vi "Update.vi"(6 "Engine in":refnum<class "Engine.lvclass">, 7 "CursorIn":refnum<class "RT_Sprite.lvclass">, 8 "error in (no error)":errorcluster, 10 "Game(readonly)":refnum<class "Game.lvclass">, 11 "GameMenu in":refnum<class "GameMenu.lvclass">) -> (0 "error out":errorcluster, 1 "State":T1, 3 "GameMenu out":refnum<class "GameMenu.lvclass">, 4 "Engine out":refnum<class "Engine.lvclass">, 5 "CursorOut":refnum<class "RT_Sprite.lvclass">)   [LabVIEW 2019, in "RT_Game.lvlib" / "GameMenu.lvclass"]
uses:
  GameMenu.lvclass
  Menu/States.ctl
  RT_Sprite/RT_Sprite.lvclass
  C:/Users/FreshBob/Dropbox/VIs/myRIO_GameConsole/RT/RT_Game/GameObject/GameObject.lvclass
  Game/Game.lvclass
  Engine/Engine.lvclass
  GameMenu.lvclass/GameMenu.ctl
  Game/Game.lvclass/Game.ctl
  Engine/Coordinate.ctl
  Engine/Engine.lvclass/Engine.ctl
  Game/Read State.vi
  Engine/Read Controls.vi
  Game/Read Singleplayer.vi
  GameObject/GameObject.lvclass
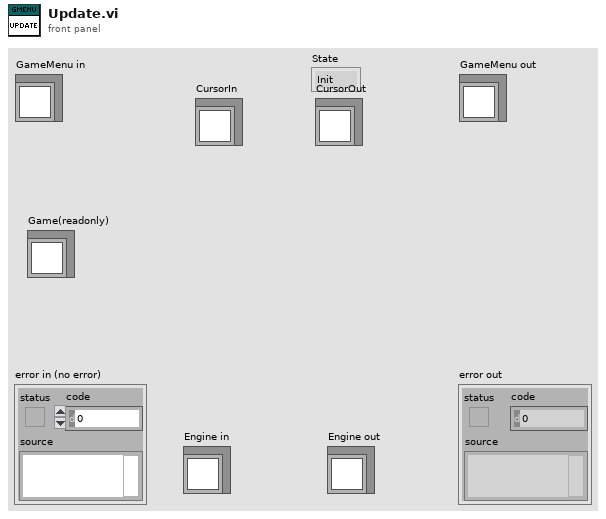
[diagram p1: front panel]
types:
  T1 = typedef "RT_Game.lvlib/Game.lvclass/States.ctl" = enum16{"Init", "Restart", "Menu", "Game", "Resume", "ToggleSingleplayer", "LoadNextGame", "ExitToMenu", "NewHighscore", "GameOver", "SlideOut", "FadeToMenu", "StartFadeToMenu"}
  T2 = typedef "RT_Game.lvlib/Engine.lvclass/Coordinate.ctl" = cluster{"x":dbl, "y":dbl}
  T3 = typedef "RT_Game.lvlib/Game.lvclass/Controls.ctl" = cluster{"Controls_1":T4, "Controls_2":cluster{"DirectionX":i8, "DirectionY":i8, "Button1":bool, "Button2":bool}, "SystemButton":bool}
  T4 = typedef "RT_Game.lvlib/Game.lvclass/ControlPlayer.ctl" = cluster{"DirectionX":i8, "DirectionY":i8, "Button1":bool, "Button2":bool}
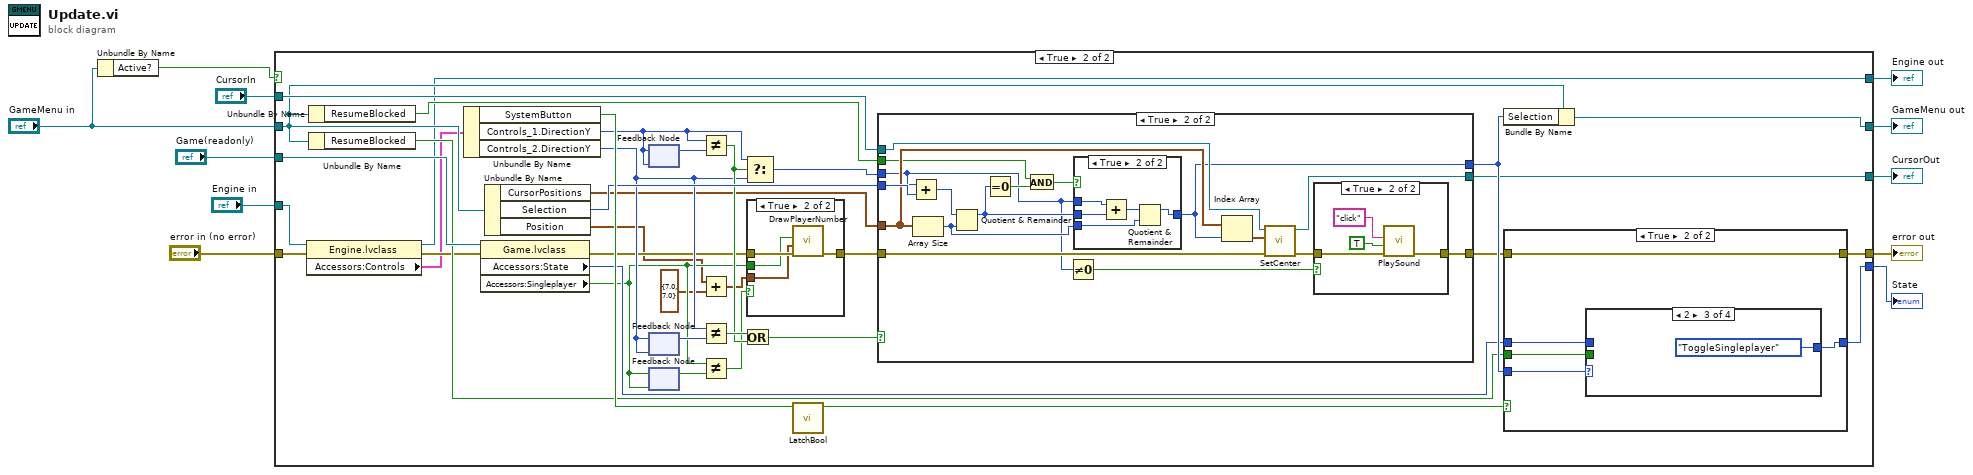
[diagram p0: block diagram]
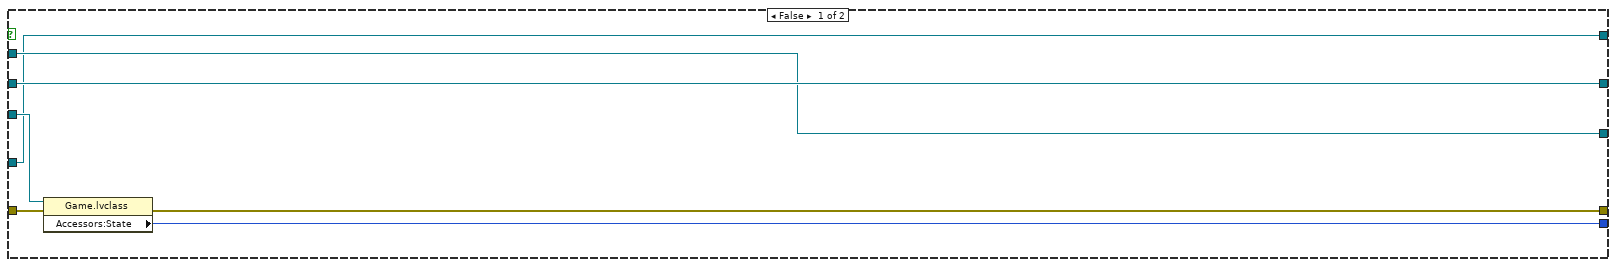
[diagram p2: hidden frame]
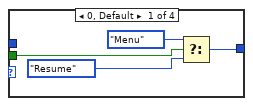
[diagram p8: hidden frame]
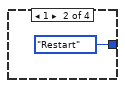
[diagram p9: hidden frame]
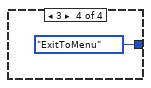
[diagram p10: hidden frame]
diagram:
  n1 = Unbundle By Name("GameMenu in") -> ("Active?"=w8:bool)
  n2 = case shown="True" w8 {
    tunnel: [w16 w54] -> w11
    tunnel: "error in (no error)" -> [w15 w40]
    tunnel: [w13 w52] -> w9
    tunnel: "GameMenu in" -> [w18 w24]
    tunnel: [w18 w36] -> w6
    tunnel: "CursorIn" -> [w17 w41]
    tunnel: [w17 w39] -> w4
    tunnel: "Game(readonly)" -> [w14 w34]
    tunnel: "Engine in" -> [w12 w21]
    tunnel: [w12 w19] -> w1
    frame False {
      n3 = property class="Game.lvclass"(reference=w14, error in=w15) -> (error out=w16:errorcluster, "Accessors:State"=w13:T1)  [unwired: 1 out]
    }
    frame True {
      n4 = property class="Engine.lvclass"(reference=w21, error in=w40) -> (reference out=w19:refnum<class "Engine.lvclass">, error out=w22:errorcluster, "Accessors:Controls"=w20:T3)
      n5 = Unbundle By Name(w24) -> ("ResumeBlocked"=w25:bool)
      n6 = Unbundle By Name(w24) -> ("ResumeBlocked"=w23:bool)
      n7 = Unbundle By Name(w20) -> ("SystemButton"=w55:bool, "Controls_1.DirectionY"=w44:i8, "Controls_2.DirectionY"=w43:i8)
      n8 = property class="Game.lvclass"(reference=w34, error in=w22) -> (error out=w35:errorcluster, "Accessors:State"=w33:T1, "Accessors:Singleplayer"=w29:bool)  [unwired: 1 out]
      n9 = Unbundle By Name(w24) -> ("CursorPositions"=w37:T2[], "Selection"=w50:i16, "Position"=w28:T2)
      n10 = feedback-in #1(w44) -> ()
      n11 = feedback #1(w44) -> (w51:i8)
      n12 = feedback #2(w43) -> (w49:i8)
      n13 = feedback-in #2(w43) -> ()
      n14 = feedback-in #3(w29) -> ()
      n15 = feedback #3(w29) -> (w32:bool)
      n16 = Not Equal?(x=w44, y=w51) -> (x != y?=w45:bool)
      n17 = Add(x=w28, y=T2 {"x"=7.0, "y"=7.0}) -> (x+y=w26:T2)
      n18 = Not Equal?(x=w43, y=w49) -> (x != y?=w47:bool)
      n19 = Not Equal?(x=w29, y=w32) -> (x != y?=w30:bool)
      n20 = Or(x=w47, y=w45) -> (x .or. y?=w48:bool)
      n21 = Select(t=w44, s=w45, f=w43) -> (s? t:f=w46:i8)
      n22 = case shown="True" w30 {
        tunnel: w35 -> [w56 w60]
        tunnel: [w56 w59] -> w31
        tunnel: w29 -> [_ w58]
        tunnel: w26 -> [_ w57]
        frame False {
        }
        frame True {
          n23 = call "DrawPlayerNumber.vi"("error in (no error)"=w60, "Position"=w57, "Accessors:Singleplayer"=w58) -> ("error out"=w59:errorcluster)  [unwired: 8 in]
        }
      }
      n24 = call "LatchBool.vi"("Boolean"=w55) -> ("Latched Boolean"=w53:bool)  [unwired: 10 in]
      n25 = case shown="True" w48 {
        tunnel: w50 -> [w63 w80]
        tunnel: [w63 w71] -> w42
        tunnel: w46 -> [_ w65]
        tunnel: w41 -> [w61 w76]
        tunnel: w31 -> [w62 w79]
        tunnel: [w61 w75] -> w39
        tunnel: [w62 w66] -> w38
        tunnel: w37 -> [_ w78]
        tunnel: w25 -> [_ w67]
        frame False {
        }
        frame True {
          n26 = Add(x=w65, y=w80) -> (x+y=w73:i16)
          n27 = Array Size(array=w78) -> (size(s)=w72:i32)
          n28 = Quotient & Remainder(x=w73, y=w72) -> (x-y*floor(x/y)=w70:i32)  [unwired: 1 out]
          n29 = Equal To 0?(x=w70) -> (x = 0?=w69:bool)
          n30 = And(x=w67, y=w69) -> (x .and. y?=w68:bool)
          n31 = Not Equal To 0?(x=w65) -> (x != 0?=w64:bool)
          n32 = case shown="True" w68 {
            tunnel: w72 -> [_ w91]
            tunnel: [w86 w90] -> w71
            tunnel: w70 -> [w86 w88]
            tunnel: w65 -> [_ w87]
            frame False {
            }
            frame True {
              n33 = Add(x=w87, y=w88) -> (x+y=w89:i32)
              n34 = Quotient & Remainder(x=w89, y=w91) -> (x-y*floor(x/y)=w90:i32)  [unwired: 1 out]
            }
          }
          n35 = Index Array(array=w78, index=w71) -> (element=w74:T2)
          n36 = call "SetCenter.vi"("error in (no error)"=w79, "center_position"=w74, "GameObject in"=w76) -> ("error out"=w77:errorcluster, "GameObject out"=w75:refnum<class "RT_Sprite.lvclass">)  [unwired: 7 in]
          n37 = case shown="True" w64 {
            tunnel: w77 -> [w81 w85]
            tunnel: [w81 w84] -> w66
            frame False {
            }
            frame True {
              n38 = call "PlaySound.vi"("error in (no error)"=w85, "Overwrite"=TRUE, "Name"="click") -> ("error out"=w84:errorcluster)  [unwired: 8 in]
            }
          }
        }
      }
      n39 = Bundle By Name(cluster=w24, "Selection"=w42) -> (w36:refnum<class "GameMenu.lvclass">)
      n40 = case shown="True" w53 {
        tunnel: w38 -> [w93 w98]
        tunnel: [w93 w98] -> w54
        tunnel: [w92 w97] -> w52
        tunnel: w33 -> [w92 w95]
        tunnel: w42 -> [_ w96]
        tunnel: w23 -> [_ w94]
        frame False {
        }
        frame True {
          n41 = case shown="2" w96 {
            tunnel: [w101 States."Restart" ("State") States."ToggleSingleplayer" ("State") States."ExitToMenu" ("State")] -> w97
            tunnel: w95 -> [_ _ _ _]
            tunnel: w94 -> [w99 _ _ _]
            frame 0, Default {
              n42 = Select(t=States."Menu", s=w99, f=States."Resume" ("State")) -> (s? t:f=w101:T1)
            }
            frame 1 {
            }
            frame 2 {
            }
            frame 3 {
            }
          }
        }
      }
    }
  }
  "error out" <- w11
  "GameMenu out" <- w6
  "State" <- w9
  "CursorOut" <- w4
  "Engine out" <- w1
